vi "countrate.vi"() -> ()   [LabVIEW 2015]
uses:
  <vilib>/Platform/TimedLoop/XDataNode/timing_clust.ctl
  <vilib>/Platform/TimedLoop/XDataNode/nitl_modes.ctl
  <vilib>/Platform/TimedLoop/XDataNode/wakeup.ctl
  <vilib>/imath/engines/lvmath2/RunTimeEngine/Managers/WorkSpace/UID Generator.vi
  <vilib>/imath/engines/lvmath2/RunTimeEngine/RunTimeType/NIMS_RunTimeType_From StrictType (excl LVString).vi
  <instcachedir>/0/NIMS_RunTimeType_From StrictType (excl LVString)_EB1C38A9BC5048DA9ABDA8F781E54D21.lvgen/NIMS_RunTimeType_From StrictType (excl LVString)_EB1C38A9BC5048DA9ABDA8F781E54D21_000.vi
  <vilib>/imath/engines/lvmath2/RunTimeEngine/LocalVariableDefStatement/MC_LocalVariableDefStatement_Display.vi
  <vilib>/imath/engines/lvmath2/RunTimeEngine/Managers/SymbolTable/Clear UID.vi
  <vilib>/imath/engines/lvmath2/RunTimeEngine/NodeEndStatement/NIMS_NodeEndStatement_Output.vi
  <instcachedir>/0/NIMS_NodeEndStatement_Output_53EC0D466D134D7ABD903AC30B43404B.lvgen/NIMS_NodeEndStatement_Output_53EC0D466D134D7ABD903AC30B43404B_010.vi
  <vilib>/imath/engines/lvmath2/RunTimeEngine/ErrorHandling/NIMS_Finalize Error.vi
  <vilib>/Utility/file.llb/Write Delimited Spreadsheet (I64).vi
  <vilib>/platform/TimedLoop/XDataNode/XDataNode.xnode
  <vilib>/Platform/TimedLoop/XDataNode/XDNodeRunTimeDep.lvlib
  <vilib>/imath/engines/lvmath2/RunTimeEngine/Managers/SymbolTable/NIMS_WorkSpace.lvlib
panel:
  in  "Total Time":dbl
  out "Waveform Graph":i32[](graph)
  in  "Period":i64=1000
  out "counts per second":dbl(knob) scale=0.0..100.0
  in  "stop":bool
  # "Demo count rate VI for Physics 434"
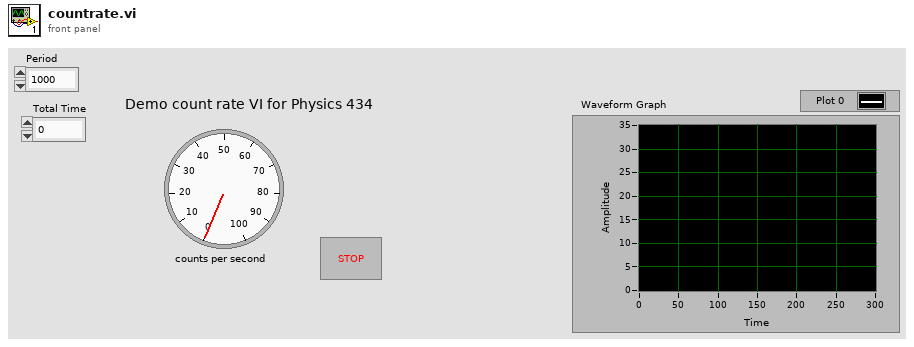
[diagram p1: front panel]
types:
  T1 = typedef "XDNodeRunTimeDep.lvlib/timing_clust.ctl" = cluster{"Expected End [f-1]":u64, "Actual End [f-1]":u64, "Finished Late? [f-1]":bool, "Expected End [i-1]":u64, "Actual End [i-1]":u64, "Finished Late? [i-1]":bool, "Expected Start [i]":u64, "Actual Start [i]":u64, "Expected Start [f]":u64, "Actual Start [f]":u64, "Source Name":string, "Structure Name":string, "Period":i64, "Deadline":i64, "Offset":i64, "Start":i64, "Priority":i32, "Timeout":i32, "Mode":T2, "Wakeup Reason":T3, "Error":errorcluster, "Source Type":string, "Secondary Source Type":string, "Global End Time":u64, "Global Start Time":u64, "Frame Duration":u64, "Iteration Duration":u64, "Assigned CPU":i32, "I/O Scan Engine Mode":u32}
  T2 = typedef "XDNodeRunTimeDep.lvlib/nitl_modes.ctl" = enum32{"No Change", "Process missed periods, maintain original phase", "Discard missed periods, maintain original phase", "Process missed periods, ignore original phase", "Discard missed periods, ignore original phase"}
  T3 = typedef "XDNodeRunTimeDep.lvlib/wakeup.ctl" = enum32{"Normal", "Aborted", "Asynchronous wakeup", "Timing source error", "Timed loop error", "Timeout"}
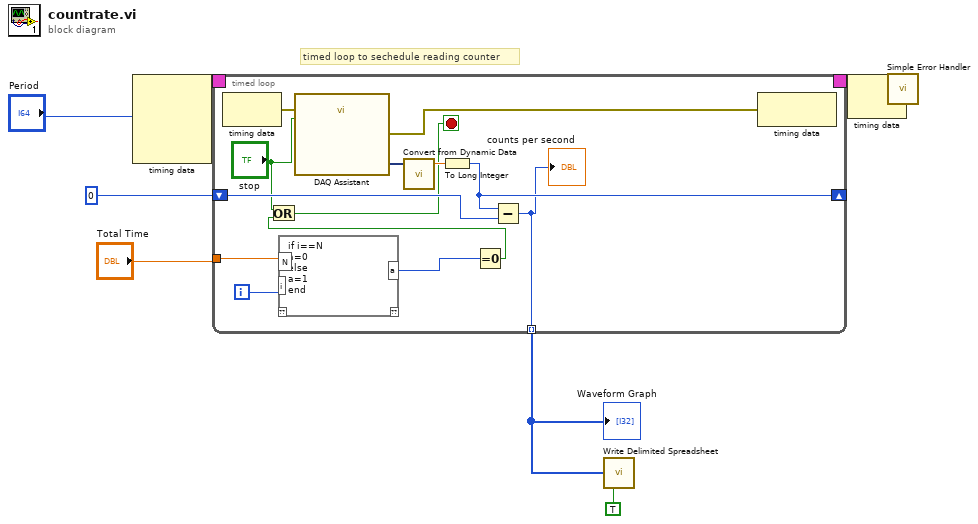
[diagram p0: block diagram]
diagram:
  # "timed loop to sechedule reading counter"
  n1 = node-c288("Period") -> (w8:T1)  [unwired: 3 in]
  n2 = timed-loop {
    timing: w8 -> [_]
    timing-out: [_] -> w7
    shift-right: [w19] -> _
    shift-left: 0 -> [w20]
    tunnel: [w15] -> w2 mode=indexing
    tunnel: "Total Time" -> [w9]
    i -> [w14]
    stop <- w11 stop-if-true
    n3 = node-c288() -> (w16:errorcluster)  [unwired: 1 in]
    n4 = mathscript code="if i==N\na=0\nelse\na=1\nend"("N"=w9, "i"=w14) -> ("a"=w13:i32)  [unwired: 1 in, 1 out]
    n5 = call "DAQ Assistant"("error in"=w16, "stop (F)"="stop") -> ("data"=w21:dynamicdata, "error out"=w17:errorcluster)  [unwired: 14 in, 2 out]
    n6 = call "Convert from Dynamic Data"("Dynamic Data Type"=w21) -> ("Scalar"=w18:dbl)  [unwired: 3 in]
    n7 = To Long Integer(number=w18) -> (32bit integer=w19:i32)
    n8 = Equal To 0?(x=w13) -> (x = 0?=w12:bool)
    n9 = Or(x="stop", y=w12) -> (x .or. y?=w11:bool)
    n10 = Subtract(x=w19, y=w20) -> (x-y=w15:i32)
    "counts per second" <- w15
    n11 = node-c288(w17) -> ()  [unwired: 1 out]
  }
  "Waveform Graph" <- w2
  n12 = call-poly <vilib>:"Write Delimited Spreadsheet.vi"("1D data"=w2, "transpose? (F)"=TRUE) -> ()  [unwired: 12 in, 2 out]
  n13 = node-c288(w7) -> (w5:errorcluster)
  n14 = call <vilib>:"Simple Error Handler.vi"("error in (no error)"=w5) -> ()  [unwired: 4 in, 5 out]
